vi "UA_GetNodenameValue.vi"(9 "node name":string, 11 "Data":string) -> (3 "value":string)   [LabVIEW 2013]
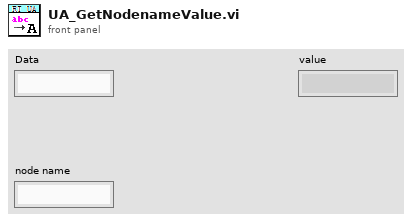
[diagram p1: front panel]
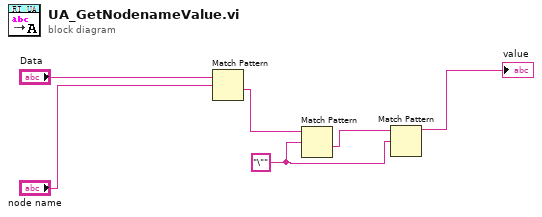
[diagram p0: block diagram]
diagram:
  w2 = "\"" ("正则表达式")
  n1 = Match Pattern(string="Data", regular expression="node name") -> (after substring=w4:string)  [unwired: 1 in, 3 out]
  n2 = Match Pattern(string=w4, regular expression=w2) -> (after substring=w3:string)  [unwired: 1 in, 3 out]
  n3 = Match Pattern(string=w3, regular expression=w2) -> (before substring=→"value":string)  [unwired: 1 in, 3 out]
